vi "load runtime from configuration.vi"(8 "error in":errorcluster, 11 "engine configuration in":T1) -> (0 "error out":errorcluster, 1 "Component Runtime Objects":refnum<class "TBM module execution interface.lvclass">[](array[class]), 2 "Engine Runtime Object":refnum<class "Engine Runtime Interface.lvclass">, 3 "engine configuration out":T1)   [LabVIEW 2013, in "PLConfigurationSerializer.lvlib"]
doc: "walks through a set of engine and module configurations and loads the matching runtime components."
uses:
  PLConfigurationSerializer.lvlib
  engines cluster.ctl
  <vilib>/NI/Module Execution Interface/Engine Configuration/engine configuration.lvclass
  <vilib>/NI/Tag Bus Module Framework/module configuration/TBM module configuration.lvclass
  <vilib>/NI/Tag Bus Module Framework/runtime/TBM module execution interface.lvclass
  <vilib>/NI/Module Execution Interface/Engine Runtime/Engine Runtime Interface.lvclass
  <vilib>/NI/CEF/CEF_TreeControl/class discovery singleton/class discovery singleton methods.ctl
  <vilib>/NI/CEF/CEF_TreeControl/class discovery singleton/class discovery singleton.lvlib
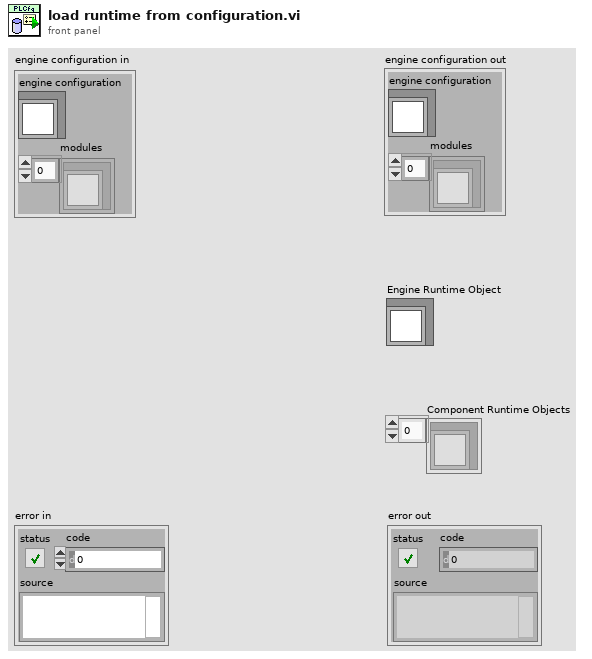
[diagram p1: front panel]
types:
  T1 = typedef "PLConfigurationSerializer.lvlib/engines cluster.ctl" = cluster{"engine configuration":refnum<class "engine configuration.lvclass">, "modules":refnum<class "TBM module configuration.lvclass">[]}
  T2 = typedef "class discovery singleton.lvlib/class discovery singleton methods.ctl" = enum16{"add search paths", "load class by name", "list available classes", "get class path"}
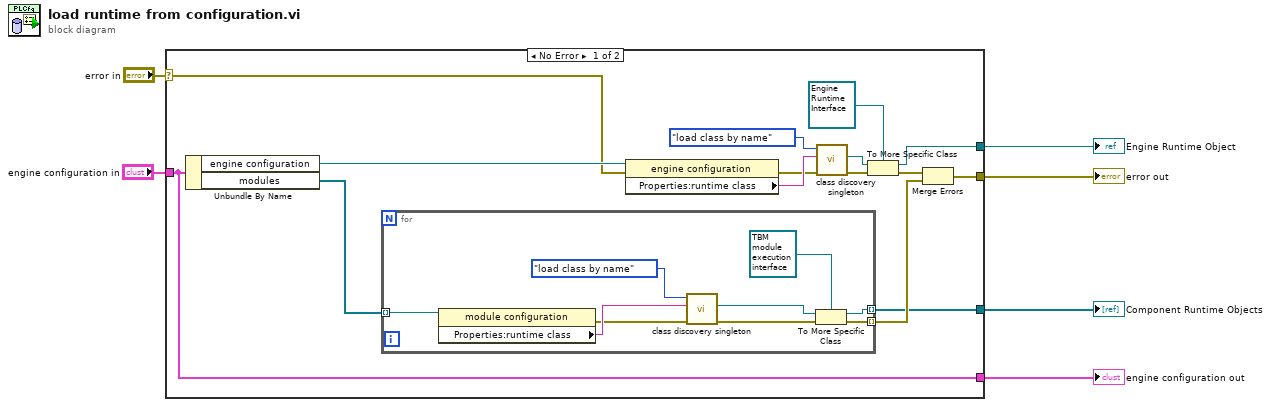
[diagram p0: block diagram]
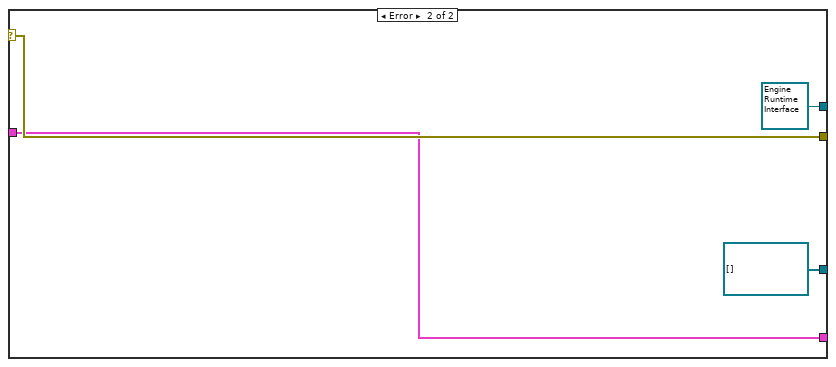
[diagram p2: hidden frame]
diagram:
  n1 = case shown="No Error" "error in" {
    selector: "error in" -> [w7 w34]
    tunnel: "engine configuration in" -> [w8 w31]
    tunnel: [w10 w34] -> w4
    tunnel: [w13 refnum<class "Engine Runtime Interface.lvclass"> refnum ("Engine Runtime Object")] -> w3
    tunnel: [w9 refnum<class "TBM module execution interface.lvclass">[] [] ("Component Runtime Objects")] -> w2
    tunnel: [w8 w31] -> w1
    frame No Error {
      n2 = Unbundle By Name(w8) -> ("engine configuration"=w20:refnum<class "engine configuration.lvclass">, "modules"=w21:refnum<class "TBM module configuration.lvclass">[])
      n3 = for {
        tunnel: w21 -> [w30] mode=indexing
        tunnel: [w23] -> w11 mode=indexing
        tunnel: [w22] -> w9 mode=indexing
        n4 = property class="module configuration"(reference=w30) -> (error out=w24:errorcluster, "Properties:runtime class"=w25:string)  [unwired: 1 in, 1 out]
        n5 = call <vilib>:"class discovery singleton.vi"("error in"=w24, "Class Name"=w25, "method"=class_discovery_singleton_methods."load class by name") -> ("error out"=w27:errorcluster, "LabVIEW Object"=w28:refnum<class>)  [unwired: 5 in, 2 out]
        n6 = To More Specific Class(target class=refnum<class "TBM module execution interface.lvclass"> refnum ("Component Runtime Interface"), reference=w28, error in=w27) -> (specific class reference=w22:refnum<class "TBM module execution interface.lvclass">, error out=w23:errorcluster)
      }
      n7 = property class="engine configuration"(reference=w20, error in=w7) -> (error out=w17:errorcluster, "Properties:runtime class"=w19:string)  [unwired: 1 out]
      n8 = call <vilib>:"class discovery singleton.vi"("error in"=w17, "Class Name"=w19, "method"=class_discovery_singleton_methods."load class by name") -> ("error out"=w16:errorcluster, "LabVIEW Object"=w15:refnum<class>)  [unwired: 5 in, 2 out]
      n9 = To More Specific Class(target class=refnum<class "Engine Runtime Interface.lvclass"> refnum ("Engine Runtime Object"), reference=w15, error in=w16) -> (specific class reference=w13:refnum<class "Engine Runtime Interface.lvclass">, error out=w12:errorcluster)
      n10 = Merge Errors(w12, w11) -> (w10:errorcluster)
    }
    frame Error {
    }
  }
  "error out" <- w4
  "Component Runtime Objects" <- w2
  "Engine Runtime Object" <- w3
  "engine configuration out" <- w1
